vi "PID控制器.vi"() -> ()   [LabVIEW 2018]
panel:
  out "实测值":dbl=-3.179097630620999e-09
  out "微控制量":dbl=1.0384162700162625e-10
  out "控制量":dbl=2.076832540032525e-09
  in  "微分系数":dbl=0.1
  in  "积分系数":dbl=0.5
  in  "比例":dbl=4.0
  out "e(k-1)":dbl=3.2101269527194835e-09 format="%.2f"
  out "e(k)":dbl=3.179097630620999e-09 format="%.2f"
  out "Waveform Chart":cluster{"Temperature":dbl, "设定值":i8, dbl, i32}(graph)={"Temperature"=-3.179097630620999e-09, "设定值"=0, 2.076832540032525e-09, 0}
  in  "设定值":i8 min=0 max=85 step=1
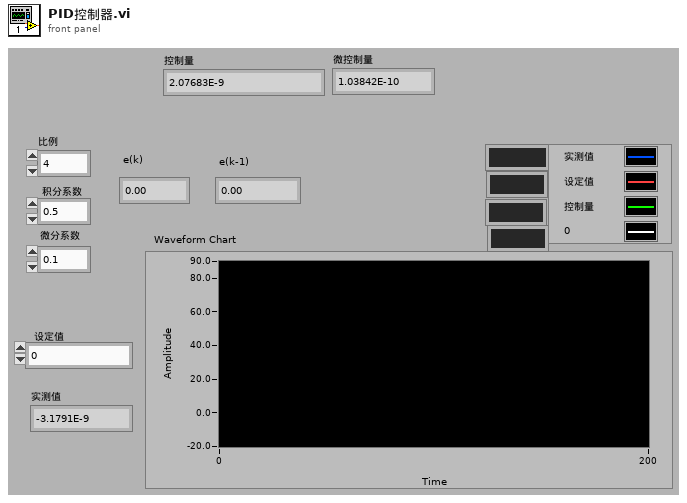
[diagram p1: front panel]
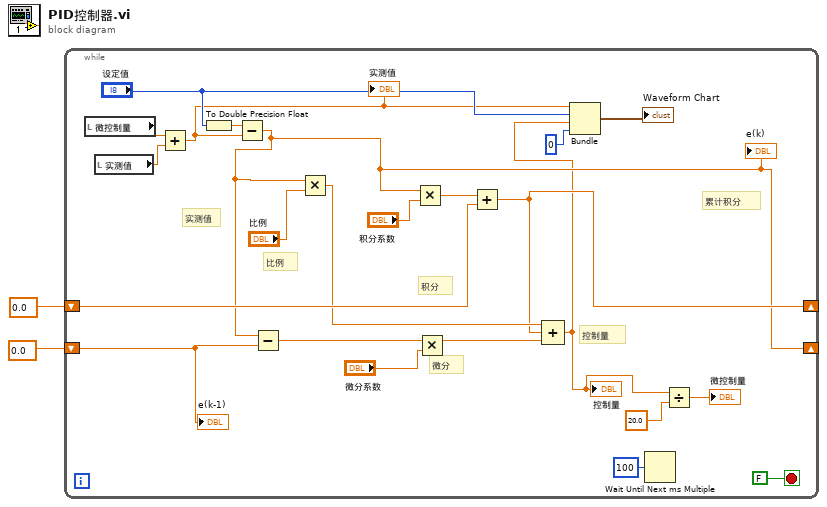
[diagram p0: block diagram]
diagram:
  n1 = while {
    shift-left: 0.0 -> [w24]
    shift-right: [w22] -> _
    shift-left: 0.0 -> [w16]
    shift-right: [w15] -> _
    stop <- FALSE stop-if-true
    # "实测值"
    # "控制量"
    # "积分"
    # "比例"
    # "微分"
    # "累计积分"
    n2 = local read "微控制量"() -> (w5:dbl)
    n3 = local read "实测值"() -> (w4:dbl)
    n4 = Add(x=w5, y=w4) -> (x+y=w6:dbl)
    "实测值" <- w6
    n5 = To Double Precision Float(number="设定值") -> (double precision float=w3:dbl)
    n6 = Subtract(x=w3, y=w6) -> (x-y=w15:dbl)
    "e(k)" <- w15
    n7 = Subtract(x=w15, y=w16) -> (x-y=w18:dbl)
    n8 = Multiply(x=w15, y="比例") -> (x*y=w23:dbl)
    n9 = Multiply(x=w15, y="积分系数") -> (x*y=w25:dbl)
    n10 = Multiply(x=w18, y="微分系数") -> (x*y=w21:dbl)
    n11 = Add(x=w25, y=w24) -> (x+y=w22:dbl)
    n12 = Compound Arithmetic op=ADD(w23, w22, w21) -> (w9:dbl)
    "控制量" <- w9
    n13 = Bundle(w6, "设定值"="设定值", w9, 0) -> (→"Waveform Chart":cluster{dbl, "设定值":i8, dbl, i32})  [unwired: 1 out]
    n14 = Wait Until Next ms Multiple(millisecond multiple=u32 100) -> ()  [unwired: 1 out]
    n15 = Divide(x=w9, y=20.0) -> (x/y=→"微控制量":dbl)
    "e(k-1)" <- w16
  }
